vi "Stop Core.vi"(10 "final error code":i32, 11 "CS++DIMMonitor in":refnum<class "CS++DIMMonitor.lvclass">) -> (3 "CS++DIMMonitor out":refnum<class "CS++DIMMonitor.lvclass">)   [LabVIEW 2016, in "CS++DIMMonitor.lvlib" / "CS++DIMMonitor.lvclass"]
doc: "(<B>Filename</B>: Actor Framework.lvlib:Actor.lvclass:Stop Core.vi)\n\nDefines what the actor does before it stops. Use the <B>final error code</B> input to determine whether the actor shut down in response to an error.\n\nBy default, this method does nothing. A descendant class may override it to define behavior, such as shutting down any processes the actor initiated in its override of the Actor Core method."
uses:
  CS++DIMMonitor.lvclass
  CS++DIMMonitor.lvclass/CS++DIMMonitor.ctl
  CSPP_Core/Actors/CS++PVMonitor/CS++PVMonitor.lvclass
  DimLVEvent/LVDimInterface/LVDimInterface.lvlib
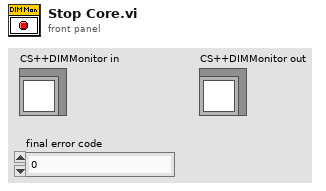
[diagram p1: front panel]
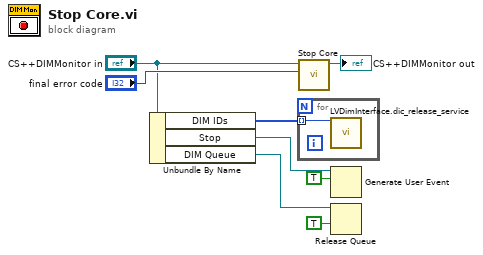
[diagram p0: block diagram]
diagram:
  n1 = Unbundle By Name("CS++DIMMonitor in") -> ("DIM IDs"=w5:i32[], "Stop"=w3:refnum<user-event>, "DIM Queue"=w2:refnum<queue>)
  n2 = for {
    tunnel: w5 -> [w9] mode=indexing
    n3 = call "LVDimInterface.dic_release_service.vi"("callBackID"=w9) -> ()  [unwired: 18 in, 1 out]
  }
  n4 = call-parent "Stop Core.vi"("final error code"="final error code", "CS++BaseActor in"="CS++DIMMonitor in") -> ("CS++BaseActor out"=→"CS++DIMMonitor out":refnum<class "CS++DIMMonitor.lvclass">)  [unwired: 9 in]
  n5 = Generate User Event(user event=w3, event data cluster=TRUE ("event data")) -> ()  [unwired: 2 in, 2 out]
  n6 = Release Queue(queue=w2, force destroy? (F)=TRUE) -> ()  [unwired: 1 in, 3 out]
